vi "Draw.vi"(8 "Error In":errorcluster, 10 "PictureIn":picture, 11 "reference in":refnum<class "Object.lvclass">) -> (0 "Error Out":errorcluster, 2 "PictureOut":picture, 3 "reference out":refnum<class "Object.lvclass">)   [LabVIEW 2020, in "Object.lvclass"]
uses:
  Object.lvclass
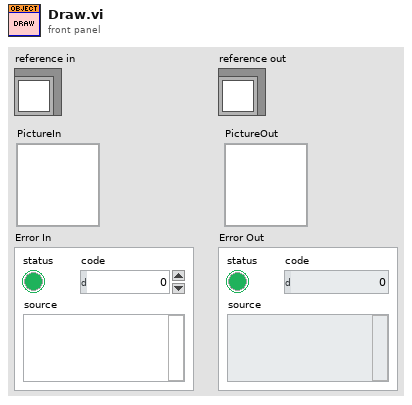
[diagram p1: front panel]
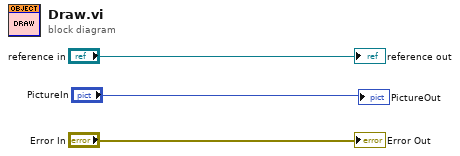
[diagram p0: block diagram]
diagram:
  "Error Out" <- "Error In"
  "reference out" <- "reference in"
  "PictureOut" <- "PictureIn"
